vi "Word_Write_Numeric_From_Bookmarks_File.vi"(4 "Bookmark Cell Range 2":string="A2", 6 "Bookmark Cell Range 1":string="A2", 7 "Bookmarks Worksheet Number":i32=1, 8 "error in (no error)":errorcluster, 9 "Excel Sheets Reference In":refnum<k7>, 10 "Bookmarks File Path":string="C:\\Teststand\\LVFiles\\Support\\Bookmarks_Table.xlsx", 11 "Word Report Reference In":refnum<class "NI_report.lvclass">) -> (0 "error out":errorcluster, 1 "Excel Sheets Reference Out":refnum<k7>, 3 "Word Report Reference Out":refnum<class "NI_report.lvclass">)   [LabVIEW 2014]
uses:
  <vilib>/Utility/NIReport.llb/NI_report.lvclass
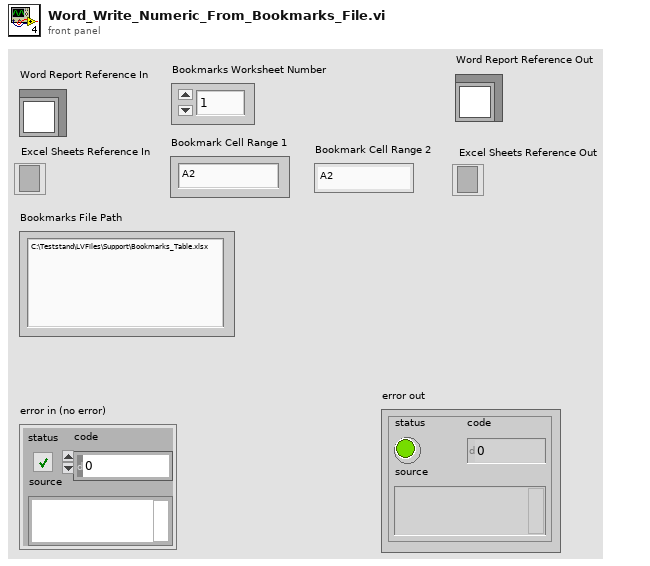
[diagram p1: front panel]
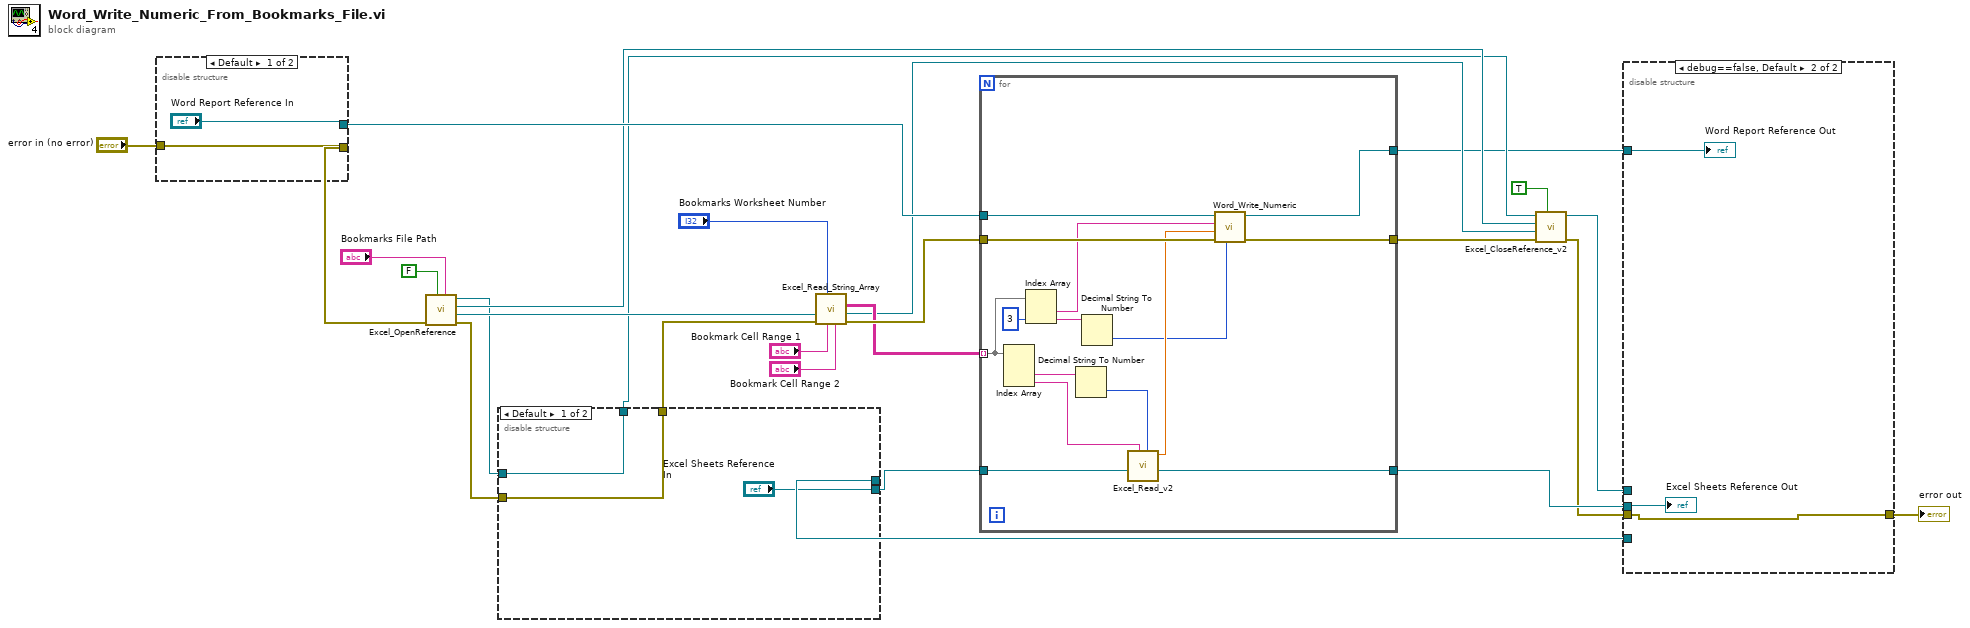
[diagram p0: block diagram]
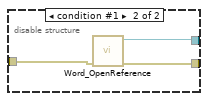
[diagram p2: hidden frame]
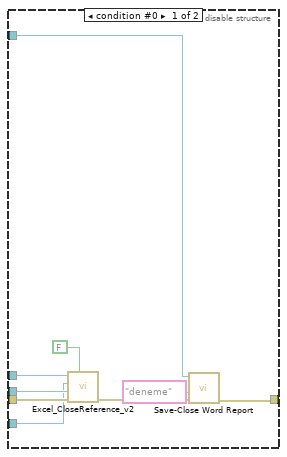
[diagram p3: hidden frame]
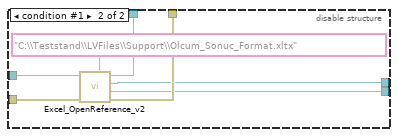
[diagram p4: hidden frame]
diagram:
  n1 = disable-structure shown="Default" {
    disable-tunnel: ["Word Report Reference In" w31] -> w26
    disable-tunnel: "error in (no error)" -> [w27 w30]
    disable-tunnel: [w27 w29] -> w3
    frame condition #0 (active) {
    }
    frame condition #1 {
      n2 = call "Word_OpenReference.vi"("error in (no error)"=w30) -> ("error out"=w29:errorcluster, "report out"=w31:refnum<class "NI_report.lvclass">)  [unwired: 9 in]
    }
  }
  n3 = call "Excel_OpenReference.vi"("Template File Path"="Bookmarks File Path", "File Visible ?"=FALSE, "error in (no error)"=w3) -> ("error out"=w11:errorcluster, "Sheets Reference Out"=w19:refnum<k7>, "Workbook Reference Out"=w14:refnum<k7>, "Excel Application Reference Out"=w13:refnum<k7>)  [unwired: 5 in]
  n4 = disable-structure shown="Default" {
    disable-tunnel: ["Excel Sheets Reference In" w37] -> w15
    disable-tunnel: w13 -> [w33 w41]
    disable-tunnel: [w33 w40] -> w12
    disable-tunnel: w11 -> [w32 w39]
    disable-tunnel: [w32 w38] -> w10
    disable-tunnel: [_ w36] -> w5
    frame condition #0 (active) {
    }
    frame condition #1 {
      n5 = call "Excel_OpenReference_v2.vi"("Template File Path"="C:\\Teststand\\LVFiles\\Support\\Olcum_Sonuc_Format.xltx", "error in (no error)"=w39, "Excel._Application"=w41) -> ("error out"=w38:errorcluster, "Sheets Reference Out"=w37:refnum<k7>, "Workbook Reference Out"=w36:refnum<k7>, "Excel Application Reference Out"=w40:refnum<k7>)  [unwired: 5 in]
    }
  }
  n6 = call "Excel_Read_String_Array.vi"("Cell Range 2"="Bookmark Cell Range 2", "Cell Range 1"="Bookmark Cell Range 1", "Worksheet Number"="Bookmarks Worksheet Number", "error in (no error)"=w10, "Sheets Reference In"=w19) -> ("error out"=w25:errorcluster, "Sheets Reference Out"=w16:refnum<k7>, "String Array"=w18:string[][])  [unwired: 4 in]
  n7 = for {
    tunnel: w26 -> [w56]
    tunnel: w25 -> [w55]
    tunnel: [w54] -> w1
    tunnel: [w53] -> w17
    tunnel: [w52] -> w8
    tunnel: w15 -> [w51]
    tunnel: w18 -> [w46] mode=indexing
    n8 = Index Array(array=w46) -> (element #2=w50:string, element #3=w49:string)  [unwired: 3 in, 1 out]
    n9 = Index Array(array=w46, index #2=3 ("index")) -> (element #1=w42:string, element #2=w44:string)  [unwired: 1 in]
    n10 = Decimal String To Number(string=w50) -> (number=w47:i32)  [unwired: 2 in, 1 out]
    n11 = Decimal String To Number(string=w44) -> (number=w43:i32)  [unwired: 2 in, 1 out]
    n12 = call "Excel_Read_v2.vi"("Worksheet Number"=w47, "Cell to Read"=w49, "Sheets Reference In"=w51) -> ("Sheets Reference Out"=w52:refnum<k7>, "Result"=w48:dbl)  [unwired: 6 in, 1 out]
    n13 = call "Word_Write_Numeric.vi"("String Precision"=w43, "error in (no error)"=w55, "Number [dbl]"=w48, "bookmark (\"\")"=w42, "report in"=w56) -> ("error out"=w53:errorcluster, "report out"=w54:refnum<class "NI_report.lvclass">)  [unwired: 5 in]
  }
  n14 = call "Excel_CloseReference_v2.vi"("Keep Excel Open ?"=TRUE, "error in (no error)"=w17, "Sheets Reference In"=w16, "Workbook Reference In"=w14, "Excel Application Reference In"=w12) -> ("error out"=w7:errorcluster, "Excel Application Reference Out"=w9:refnum<k7>)  [unwired: 5 in]
  n15 = disable-structure shown="debug==false, Default" {
    disable-tunnel: w9 -> [w65 _]
    disable-tunnel: [w59 w67] -> w2
    disable-tunnel: w8 -> [w63 w68]
    disable-tunnel: w7 -> [w62 w67]
    disable-tunnel: w5 -> [w61 _]
    disable-tunnel: w1 -> [w58 w66]
    frame condition #0 {
      n16 = call "Excel_CloseReference_v2.vi"("Keep Excel Open ?"=FALSE, "error in (no error)"=w62, "Sheets Reference In"=w63, "Workbook Reference In"=w61, "Excel Application Reference In"=w65) -> ("error out"=w60:errorcluster)  [unwired: 5 in, 1 out]
      n17 = call "Save-Close Word Report.vi"("error in (no error)"=w60, "Certificate File Name"="deneme", "report in"=w58) -> ("error out"=w59:errorcluster)  [unwired: 8 in]
    }
    frame condition #1 (active) {
      "Excel Sheets Reference Out" <- w68
      "Word Report Reference Out" <- w66
    }
  }
  "error out" <- w2
